vi "SQLite Insert or Update SensorConfigValue.vi"(7 "Main":string="0", 8 "error in (no error)":errorcluster, 9 "SensorConfigList":string, 11 "SensorName":string) -> (0 "error out":errorcluster, 3 "OK？":bool)   [LabVIEW 2017, in "SQLite.lvclass"]
doc: "保存传感器配置到Calibration.db.\n2020-03-06 09:56:51\n蒋松\njiangsong@outlook.com"
uses:
  SQLite.lvclass
  SQLiteFileName.ctl
  TabelFullName.ctl
  <vilib>/Utility/error.llb/Trim Whitespace.vi
  <userlib>/sushu/sushu.lvlib
  <userlib>/LabSQL/LabSQL.lvlib
panel:
  out "Insert DB String":string
  out "Insert DB String 2":string
  out "empty?":bool
  out "Select SQL CMD":string
  out "String":string
  in  "error in (no error) 2":errorcluster
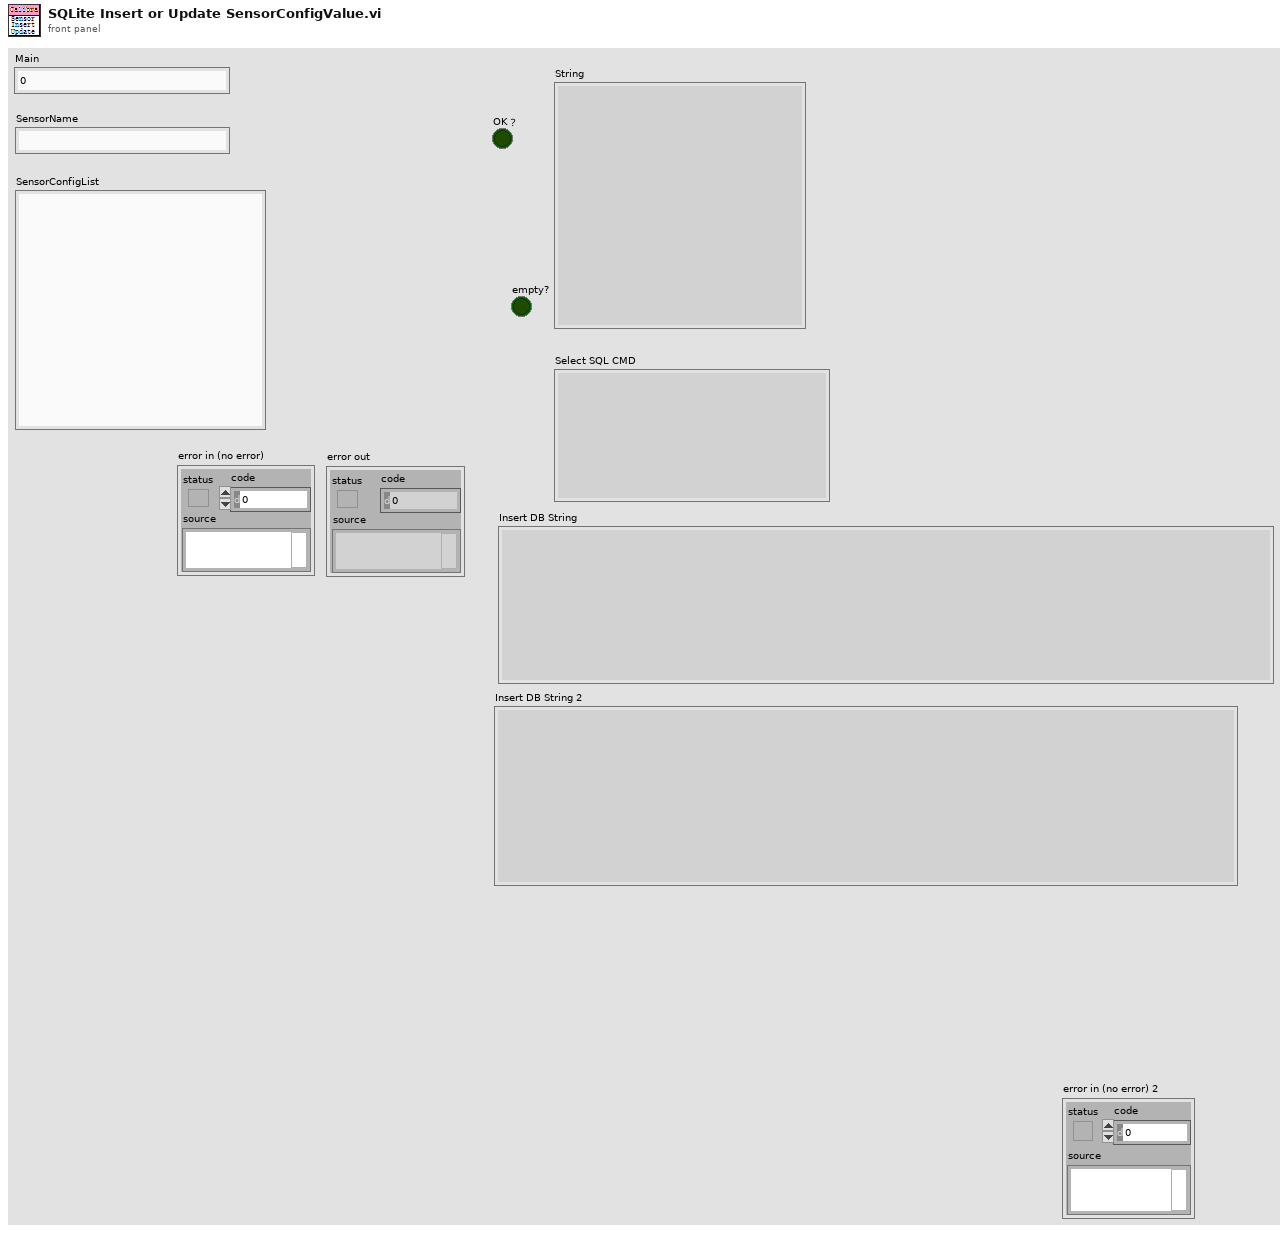
[diagram p1: front panel]
types:
  T1 = typedef "SQLite.lvclass/TabelFullName.ctl" = string
  T2 = typedef "SQLite.lvclass/SQLiteFileName.ctl" = string
  T3 = enum16{"Other", "SQL2008", "SQLite", "Access", "MySQL"}
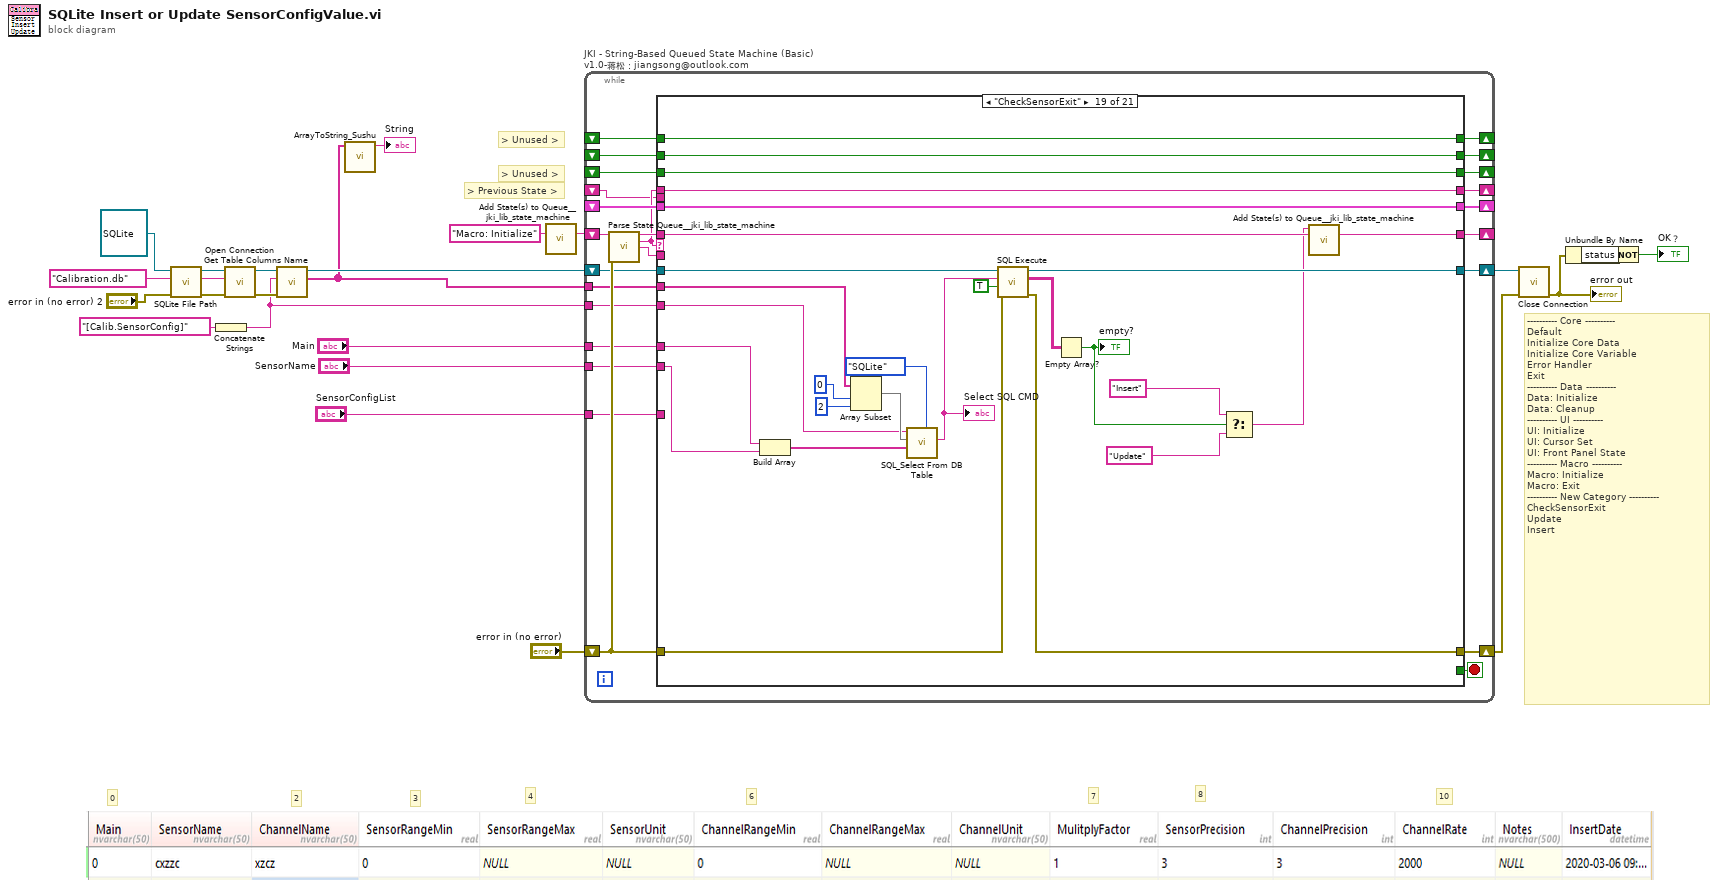
[diagram p0: block diagram]
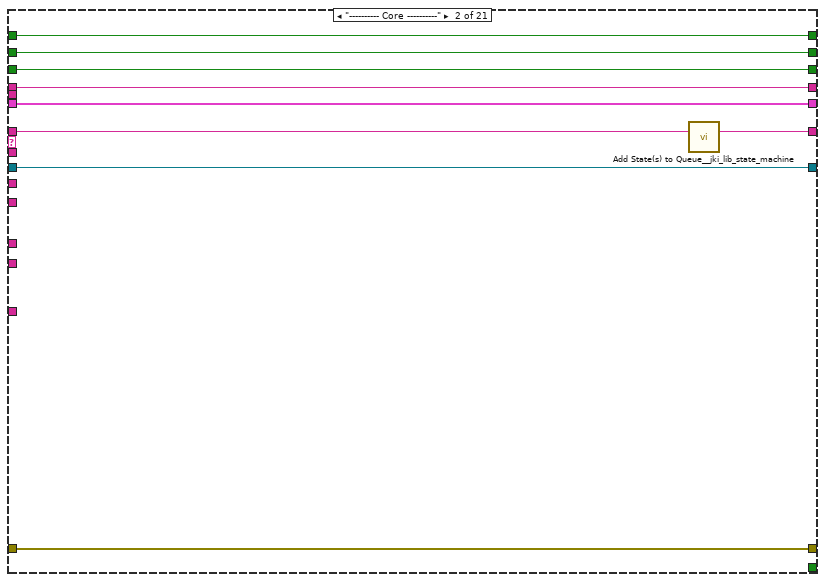
[diagram p3: hidden frame]
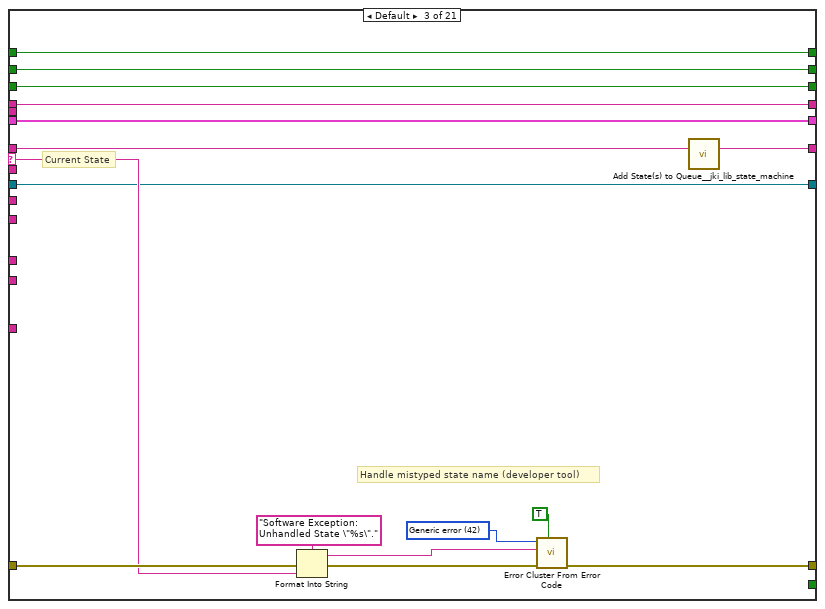
[diagram p4: hidden frame]
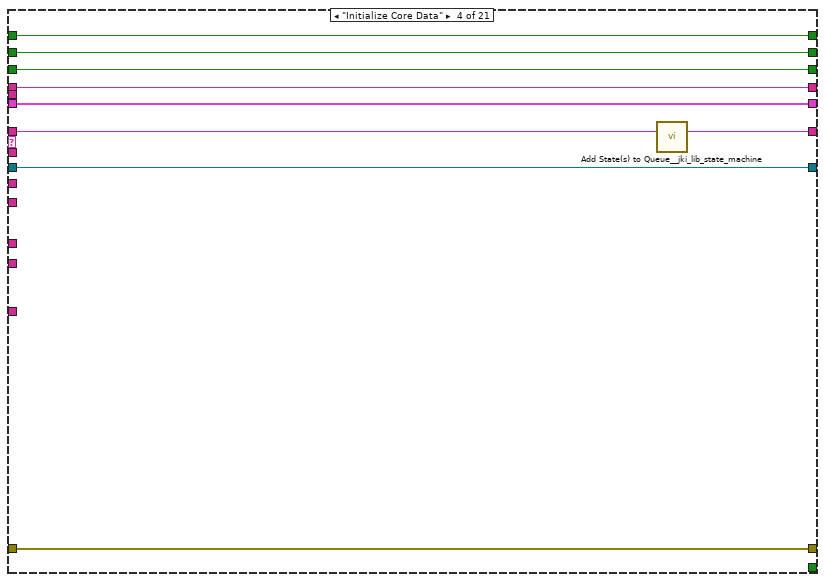
[diagram p5: hidden frame]
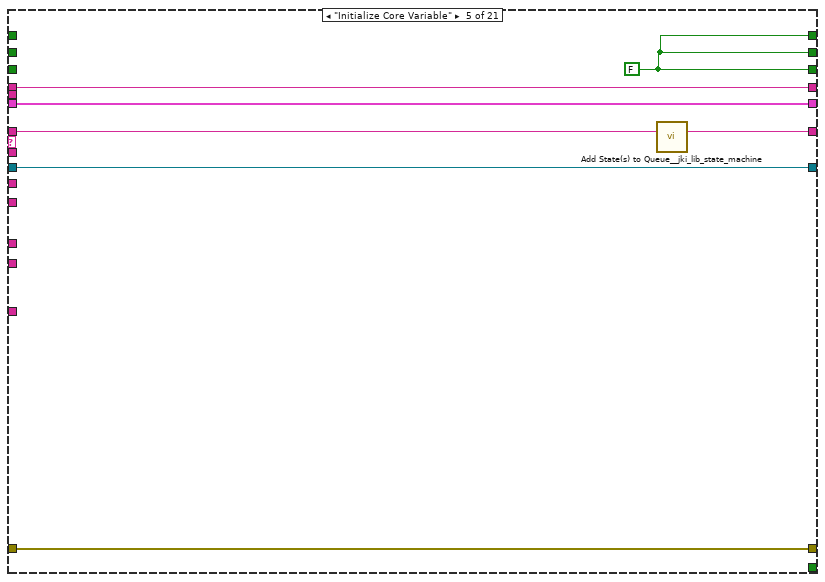
[diagram p6: hidden frame]
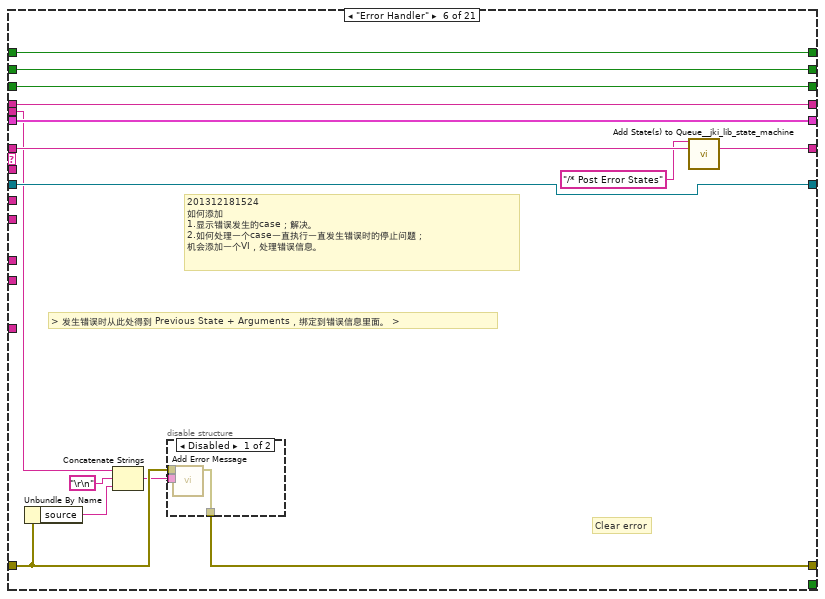
[diagram p7: hidden frame]
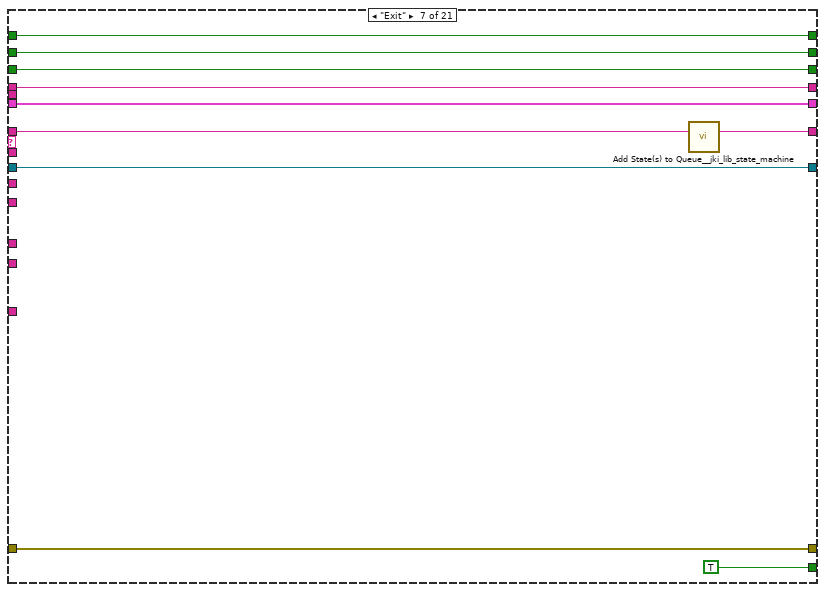
[diagram p9: hidden frame]
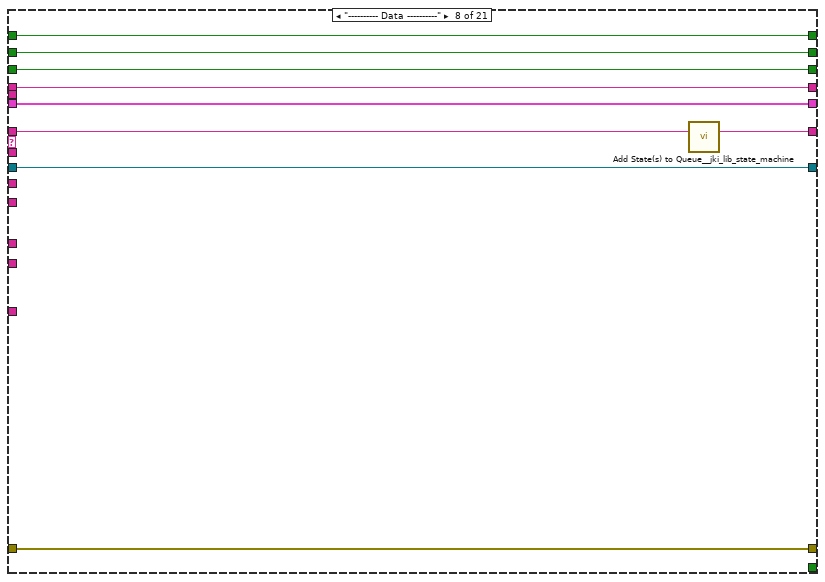
[diagram p10: hidden frame]
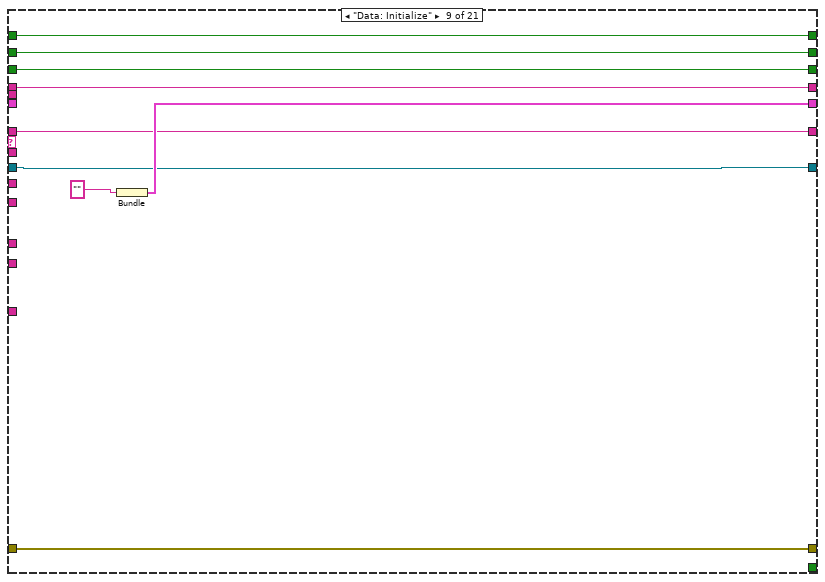
[diagram p11: hidden frame]
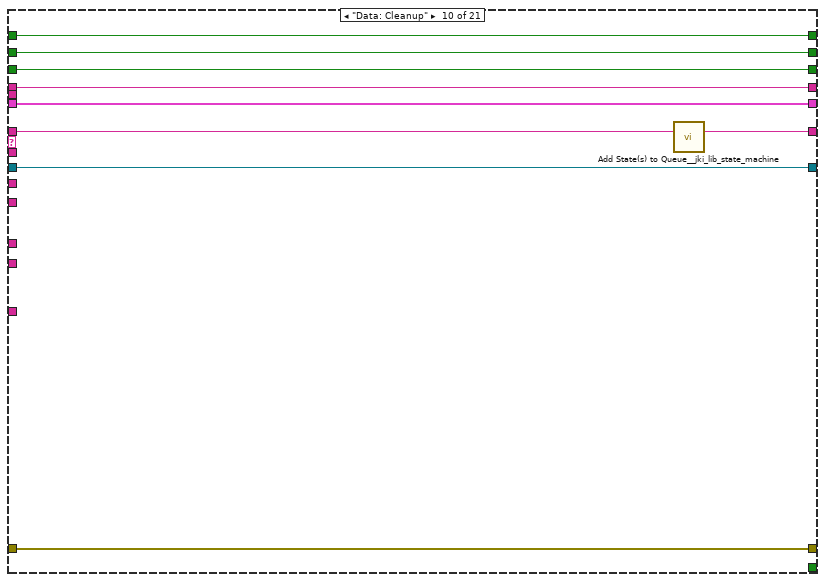
[diagram p12: hidden frame]
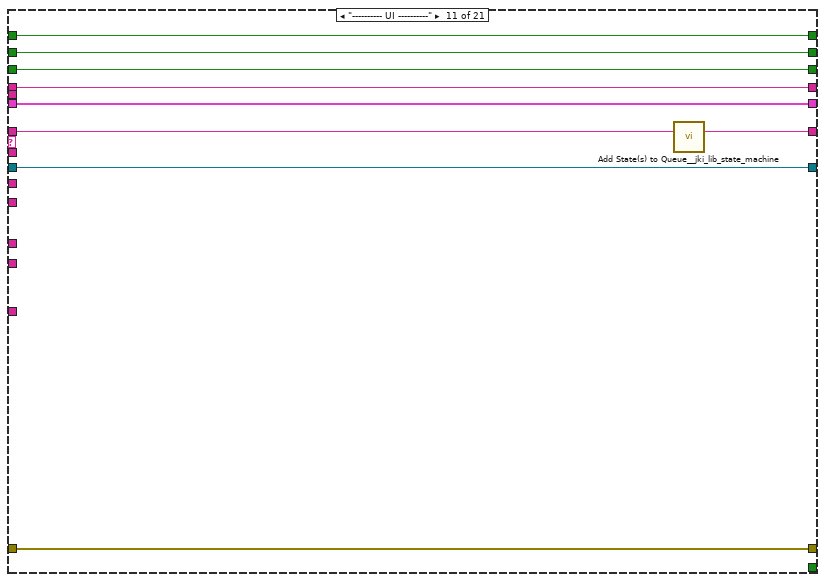
[diagram p13: hidden frame]
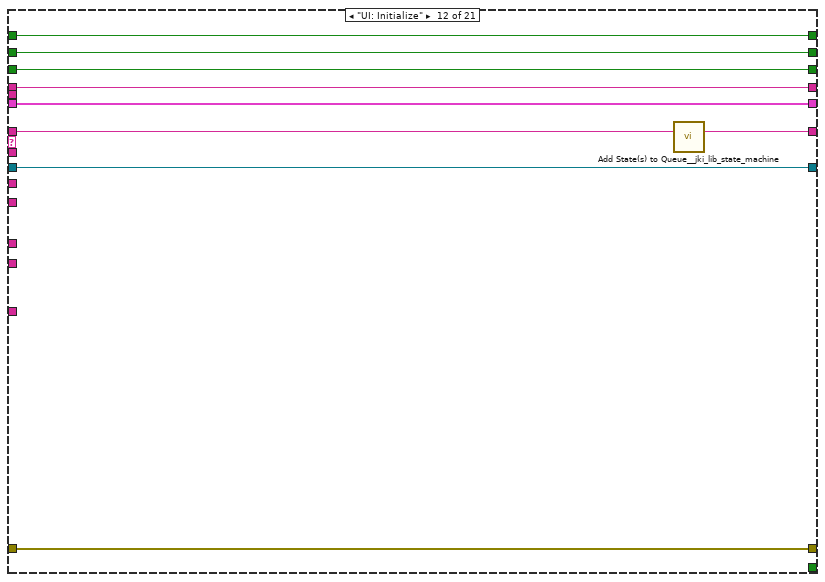
[diagram p14: hidden frame]
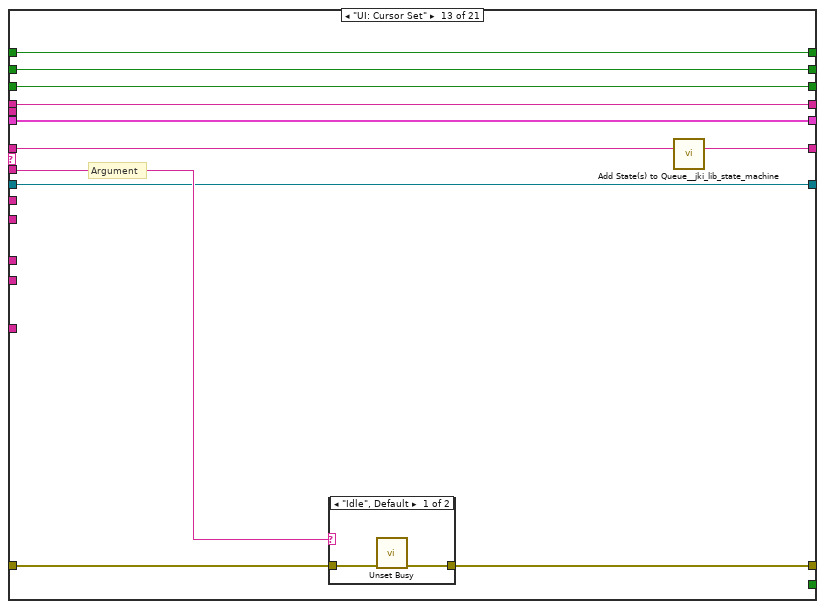
[diagram p15: hidden frame]
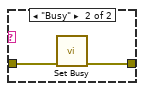
[diagram p16: hidden frame]
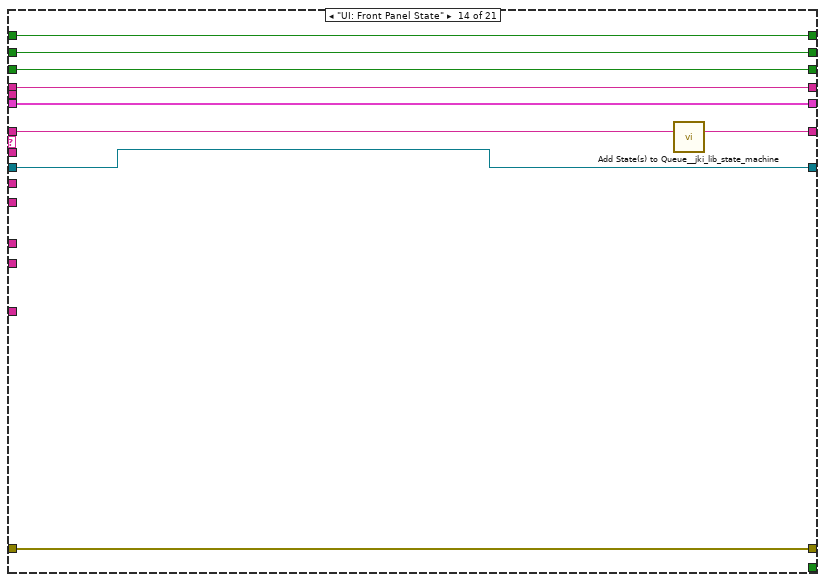
[diagram p17: hidden frame]
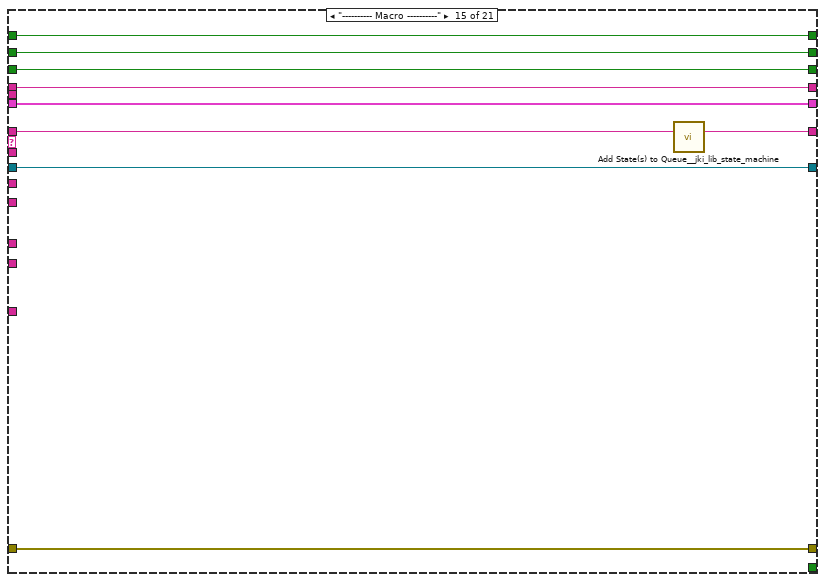
[diagram p18: hidden frame]
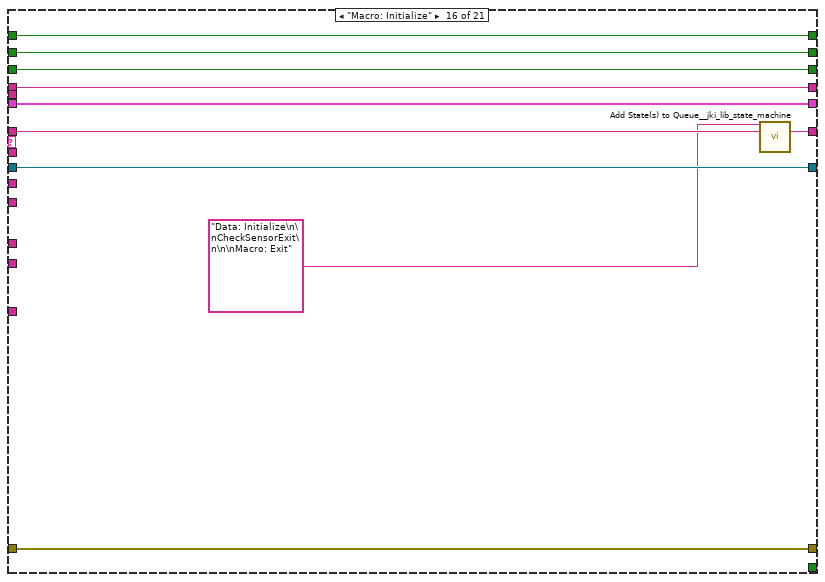
[diagram p19: hidden frame]
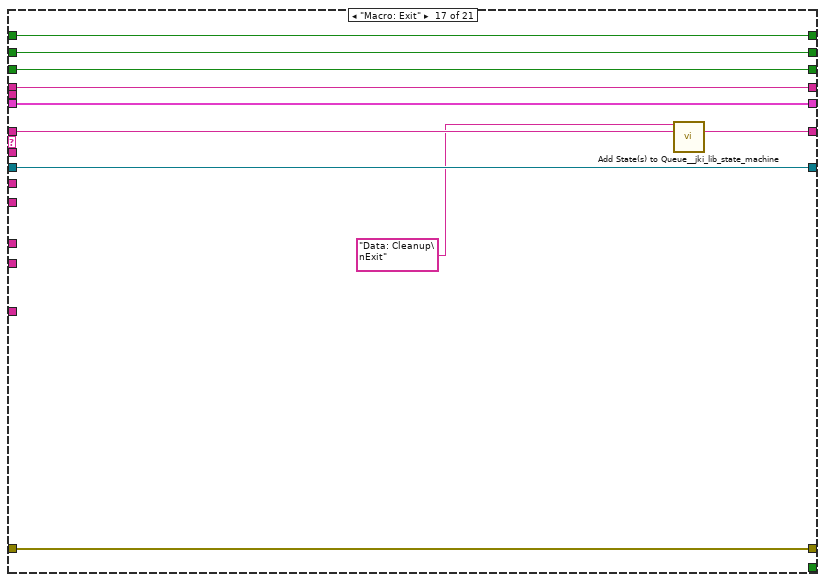
[diagram p20: hidden frame]
diagram:
  # "10"
  # "8"
  # "7"
  # "6"
  # "3"
  # "0"
  # "> Previous State >"
  # "> Unused >"
  # "> Unused >"
  # "---------- Core ----------\nDefault\nInitialize Core Data\nInitialize Core Variable\nError Handler\nExit\n---------- Data ----------\nData: Initialize\nData: Cleanup\n---------- UI ----------\nUI: Initialize\nUI: Cursor Set\nUI: Front Panel State\n---------- Macro ----------\nMacro: Initialize\nMacro: Exit\n---------- New Category ----------\nCheckSensorExit\nUpdate\nInsert"
  # "2"
  # "4"
  n1 = call "SQLite File Path.vi"("error in (no error)"="error in (no error) 2", "SQLiteFileName"=T2 "Calibration.db", "SQLite in"=refnum<class "SQLite.lvclass"> refnum ("SQLite.lvclass")) -> ("error out"=w19:errorcluster, "string"=w15:string, "SQLite out"=w17:refnum<class "SQLite.lvclass">)  [unwired: 6 in]
  n2 = Concatenate Strings(T1 "[Calib.SensorConfig]" ("TabelFullName")) -> (w10:string)
  n3 = call-dynamic "Open Connection.vi"("error in (no error)"=w19, "ConnectionString"=w15, "HostDB in"=w17) -> ("error out"=w14:errorcluster, "HostDB out"=w13:refnum<class "SQLite.lvclass">)  [unwired: 7 in]
  n4 = call-dynamic "Get Table Columns Name.vi"("error in (no error)"=w14, "TableName"=w10, "HostDB in"=w13) -> ("ColunmsList"=w6:string[], "HostDB out"=w11:refnum<class "SQLite.lvclass">)  [unwired: 4 in, 3 out]
  n5 = call <userlib>:"ArrayToString_Sushu.vi"("Array"=w6) -> ("String"=→"String":string)  [unwired: 10 in]
  n6 = call <vilib>:"Add State(s) to Queue__jki_lib_state_machine.vi"("State(s) in (\"\")"="Macro: Initialize") -> ("States Out"=w24:string)  [unwired: 14 in]
  n7 = while "JKI - String-Based Queued State Machine (Basic) v1.0-蒋松：jiangsong@outlook.com" {
    shift-right: [w47] -> w7
    shift-left: "error in (no error)" -> [w45]
    shift-right: [w28] -> _
    shift-left: w24 -> [w35]
    shift-right: [w41] -> _
    shift-left: _ -> [w43]
    shift-right: [w42] -> _
    shift-left: _ -> [w44]
    shift-right: [w36] -> _
    shift-left: _ -> [w39]
    shift-right: [w37] -> _
    shift-left: _ -> [w25]
    shift-right: [w38] -> _
    shift-left: _ -> [w40]
    tunnel: w6 -> [w34]
    tunnel: w10 -> [w33]
    tunnel: "Main" -> [w32]
    tunnel: "SensorName" -> [w31]
    shift-right: [w29] -> w9
    shift-left: w11 -> [w30]
    tunnel: "SensorConfigList" -> [w27]
    stop <- w46 stop-if-true
    n8 = call <vilib>:"Parse State Queue__jki_lib_state_machine.vi"("State Queue"=w35, "Error In (no error)"=w45) -> ("Remaining States"=w49:string, "Current State"=w26:string, "Arguments"=w48:string)  [unwired: 10 in, 1 out]
    n9 = case shown="\"CheckSensorExit\"" w26 {
      selector: w26 -> [_ _ w68 _ _ _ _ _ _ _ _ _ _ _ _ _ _ _ _ _ _]
      tunnel: w49 -> [w50 w66 w82 w91 w98 w113 w126 w135 w136 w153 w162 w171 w182 w195 w204 w206 w224 w233 w239 w283 w311]
      tunnel: w48 -> [_ _ _ _ _ _ _ _ _ _ _ _ w176 _ _ _ _ _ _ _ _]
      tunnel: [w57 w64 w69 w86 w96 w100 w119 w129 w141 w145 w156 w165 w174 w187 w198 w210 w219 w228 w236 w261 w285] -> w47
      tunnel: w45 -> [w57 w64 w70 w86 w96 w103 w119 w129 w141 w145 w156 w165 w175 w187 w198 w210 w219 w228 w237 w262 w286]
      tunnel: [w50 w65 w81 w90 w97 w112 w125 w134 w136 w152 w161 w170 w181 w194 w203 w207 w223 w232 w240 w283 w311] -> w28
      tunnel: [_ _ _ _ _ _ TRUE _ _ _ _ _ _ _ _ _ _ _ _ _ _] -> w46
      tunnel: w44 -> [w56 w63 w80 w89 _ w111 w124 w133 w144 w151 w160 w169 w180 w193 w202 w214 w222 w231 w260 w282 w310]
      tunnel: w43 -> [w55 w62 w79 w88 _ w110 w123 w132 w143 w150 w159 w168 w179 w192 w201 w213 w221 w230 w259 w281 w309]
      tunnel: [w56 w63 w80 w89 w93 w111 w124 w133 w144 w151 w160 w169 w180 w193 w202 w214 w222 w231 w260 w282 w310] -> w42
      tunnel: [w55 w62 w79 w88 w93 w110 w123 w132 w143 w150 w159 w168 w179 w192 w201 w213 w221 w230 w259 w281 w309] -> w41
      tunnel: w40 -> [w54 w61 w78 w87 _ w109 w122 w131 w142 w149 w158 w167 w178 w191 w200 w212 w220 w229 w258 w280 w308]
      tunnel: w26 -> [w52 w59 w77 w85 w92 w106 w118 w128 w139 w147 w155 w164 w173 w189 w197 w209 w217 w226 w257 w279 w307]
      tunnel: w39 -> [w53 w60 w76 w83 w95 w101 w121 w130 _ w148 w157 w166 w177 w190 w199 w211 w218 w227 w256 w278 w306]
      tunnel: [w54 w61 w78 w87 w93 w109 w122 w131 w142 w149 w158 w167 w178 w191 w200 w212 w220 w229 w258 w280 w308] -> w38
      tunnel: [w52 w59 w77 w85 w92 w106 w118 w128 w139 w147 w155 w164 w173 w189 w197 w209 w217 w226 w257 w279 w307] -> w37
      tunnel: [w53 w60 w76 w83 w95 w101 w121 w130 w140 w148 w157 w166 w177 w190 w199 w211 w218 w227 w256 w278 w306] -> w36
      tunnel: w34 -> [_ _ _ _ _ _ _ _ _ _ _ _ _ _ _ _ _ _ w247 w270 w292]
      tunnel: w33 -> [_ _ _ _ _ _ _ _ _ _ _ _ _ _ _ _ _ _ w246 w272 w299]
      tunnel: w32 -> [_ _ _ _ _ _ _ _ _ _ _ _ _ _ _ _ _ _ w245 w277 w305]
      tunnel: w31 -> [_ _ _ _ _ _ _ _ _ _ _ _ _ _ _ _ _ _ w244 w276 w304]
      tunnel: w30 -> [w51 w58 w67 w84 w94 w104 w117 w127 w138 w146 w154 w163 w172 w188 w196 w208 w216 w225 w249 w275 w303]
      tunnel: [w51 w58 w67 w84 w94 w104 w117 w127 w138 w146 w154 w163 w172 w188 w196 w208 w216 w225 w248 w274 w302] -> w29
      tunnel: w27 -> [_ _ _ _ _ _ _ _ _ _ _ _ _ _ _ _ _ _ _ w267 w296]
      tunnel: w25 -> [_ _ _ _ _ w99 _ _ _ _ _ _ _ _ _ _ _ _ _ _ _]
      frame "Idle" {
      }
      frame "---------- Core ----------" {
        n10 = call <vilib>:"Add State(s) to Queue__jki_lib_state_machine.vi"("State(s) in (\"\")"=w66) -> ("States Out"=w65:string)  [unwired: 14 in]
      }
      frame Default {
        w72 = 42 items=["No error", "Argument error", "Memory is full", "Out of zone", "End of file", "File already open", "Generic file I/O error", "File not found", "File permission error", "Disk is full", "Duplicate path", "Too many files open", "System feature not enabled", "Resource file not found", "Cannot add resource", "Resource not found", "Image not found", "Image memory error", "Pen does not exist", "Config type invalid", "Config token not found", "Config parse error", "Config memory error", "Bad external code format", "Bad external code offset", "External code not present", "Null window", "Destroy window error", "Null menu", "Print aborted", "Bad print record", "Print driver error", "Windows error during printing", "Memory error during printing", "Print dialog error", "Generic print error", "Invalid device refnum", "Device not found", "Device parameter error", "Device unit error", "Cannot open device", "Device call aborted", "Generic error", "Cancelled by user", "Object ID too low", "Object ID too high", "Object not in heap", "Unknown heap", "Unknown object (invalid DefProc)", "Unknown object (DefProc not in table)", "Message out of range", "Invalid (null) method", "Unknown message", "Manager call not supported", "Bad address", "Network operation in progress", "Network operation timed out", "Connection is busy", "Network attribute not supported", "Network error", "Address in use", "System out of memory", "Connection aborted", "Connection refused", "Not connected", "Already connected", "Connection closed", "Initialization error (interapplication manager)", "Bad occurrence", "Wait on unbound occurrence handler", "Occurrence queue overflow", "Datalog type conflict", "Unused", "Unrecognized type (interapplication manager)", "Memory corrupt", "Failed to make temporary DLL", "Old CIN version", "Drag socket not found", "Failed to load drop-object", "Failed to register OLE object", "Failed to release OLE object", "Format specifier type mismatch", "Unknown format specifier", "Too few format specifiers", "Too many format specifiers", "Scan failed", "Newer CIN version", "Error converting to variant", "Runtime menu error", "Password tampered", "Variant attribute not found", "Incompatible variant data type", "Event data is not available", "Event Store is not present", "Occurrence is not found", "Event Queue is not created", "Event info is not available", "Refnum passed is NULL", "Error retrieving Class GUID", "Error retrieving CoClass GUID", "Error retrieving TypeLib GUID.", "Bad built application magic bytes.", "Specific driver is different from the specific driver associated with the Logical Name.", "There is no session opened to the class driver.", "Max Error", "MAX - Error with config objects", "MAX - Error loading configuration", "MAX - Group not supported"]
        # "Current State"
        # "Handle mistyped state name (developer tool)"
        n11 = Format Into String(format string="Software Exception: Unhandled State \"%s\"." ("message"), error in=w70, w68) -> (resulting string=w73:string, error out=w74:errorcluster)  [unwired: 1 in]
        n12 = call <vilib>:"Error Cluster From Error Code.vi"("show call chain? (False)"=TRUE, "error in (no error)"=w74, "error message (\"\")"=w73, "error code (0)"=w72) -> ("error out"=w69:errorcluster)  [unwired: 5 in]
        n13 = call <vilib>:"Add State(s) to Queue__jki_lib_state_machine.vi"("State(s) in (\"\")"=w82) -> ("States Out"=w81:string)  [unwired: 14 in]
      }
      frame "Initialize Core Data" {
        n14 = call <vilib>:"Add State(s) to Queue__jki_lib_state_machine.vi"("State(s) in (\"\")"=w91) -> ("States Out"=w90:string)  [unwired: 14 in]
      }
      frame "Initialize Core Variable" {
        w93 = FALSE
        n15 = call <vilib>:"Add State(s) to Queue__jki_lib_state_machine.vi"("State(s) in (\"\")"=w98) -> ("States Out"=w97:string)  [unwired: 14 in]
      }
      frame "Error Handler" {
        # "> 发生错误时从此处得到 Previous State + Arguments，绑定到错误信息里面。 >"
        # "201312181524\n如何添加\n1.显示错误发生的case；解决。\n2.如何处理一个case一直执行一直发生错误时的停止问题；\n机会添加一个VI，处理错误信息。"
        # "Clear error"
        n16 = Unbundle By Name(w103) -> ("source"=w105:string)
        n17 = Concatenate Strings(w99, "\r\n", w105) -> (w102:string)
        n18 = disable-structure shown="Disabled" {
          disable-tunnel: w103 -> [w116 _]
          disable-tunnel: w102 -> [w115 _]
          disable-tunnel: [w114 _] -> w100
          frame Disabled {
            n19 = call <userlib>:"Add Error Message.vi"("ErrorMessages"=w115, "error in (no error)"=w116) -> ("error out"=w114:errorcluster)  [unwired: 9 in]
          }
          frame Enabled {
          }
        }
        n20 = call <vilib>:"Add State(s) to Queue__jki_lib_state_machine.vi"("State(s) in Front (\"\")"="/* Post Error States", "State(s) in (\"\")"=w113) -> ("States Out"=w112:string)  [unwired: 13 in]
      }
      frame "Exit" {
        n21 = call <vilib>:"Add State(s) to Queue__jki_lib_state_machine.vi"("State(s) in (\"\")"=w126) -> ("States Out"=w125:string)  [unwired: 14 in]
      }
      frame "---------- Data ----------" {
        n22 = call <vilib>:"Add State(s) to Queue__jki_lib_state_machine.vi"("State(s) in (\"\")"=w135) -> ("States Out"=w134:string)  [unwired: 14 in]
      }
      frame "Data: Initialize" {
        n23 = Bundle("") -> (w140:cluster{string})  [unwired: 1 in]
      }
      frame "Data: Cleanup" {
        n24 = call <vilib>:"Add State(s) to Queue__jki_lib_state_machine.vi"("State(s) in (\"\")"=w153) -> ("States Out"=w152:string)  [unwired: 14 in]
      }
      frame "---------- UI ----------" {
        n25 = call <vilib>:"Add State(s) to Queue__jki_lib_state_machine.vi"("State(s) in (\"\")"=w162) -> ("States Out"=w161:string)  [unwired: 14 in]
      }
      frame "UI: Initialize" {
        n26 = call <vilib>:"Add State(s) to Queue__jki_lib_state_machine.vi"("State(s) in (\"\")"=w171) -> ("States Out"=w170:string)  [unwired: 14 in]
      }
      frame "UI: Cursor Set" {
        # "Argument"
        n27 = case shown="\"Idle\", Default" w176 {
          tunnel: w175 -> [w184 w186]
          tunnel: [w183 w185] -> w174
          frame "Idle", Default {
            n28 = call <vilib>:"Unset Busy.vi"("error in (no error)"=w184) -> ("error out"=w183:errorcluster)  [unwired: 10 in]
          }
          frame "Busy" {
            n29 = call <vilib>:"Set Busy.vi"("error in (no error)"=w186) -> ("error out"=w185:errorcluster)  [unwired: 9 in, 1 out]
          }
        }
        n30 = call <vilib>:"Add State(s) to Queue__jki_lib_state_machine.vi"("State(s) in (\"\")"=w182) -> ("States Out"=w181:string)  [unwired: 14 in]
      }
      frame "UI: Front Panel State" {
        n31 = call <vilib>:"Add State(s) to Queue__jki_lib_state_machine.vi"("State(s) in (\"\")"=w195) -> ("States Out"=w194:string)  [unwired: 14 in]
      }
      frame "---------- Macro ----------" {
        n32 = call <vilib>:"Add State(s) to Queue__jki_lib_state_machine.vi"("State(s) in (\"\")"=w204) -> ("States Out"=w203:string)  [unwired: 14 in]
      }
      frame "Macro: Initialize" {
        n33 = call <vilib>:"Add State(s) to Queue__jki_lib_state_machine.vi"("State(s) in Front (\"\")"="Data: Initialize\n\nCheckSensorExit\n\n\nMacro: Exit", "State(s) in (\"\")"=w206) -> ("States Out"=w207:string)  [unwired: 13 in]
      }
      frame "Macro: Exit" {
        n34 = call <vilib>:"Add State(s) to Queue__jki_lib_state_machine.vi"("State(s) in Front (\"\")"="Data: Cleanup\nExit", "State(s) in (\"\")"=w224) -> ("States Out"=w223:string)  [unwired: 13 in]
      }
      frame "---------- New Category ----------" {
        n35 = call <vilib>:"Add State(s) to Queue__jki_lib_state_machine.vi"("State(s) in (\"\")"=w233) -> ("States Out"=w232:string)  [unwired: 14 in]
      }
      frame "CheckSensorExit" {
        n36 = Build Array(w245, w244) -> (w253:string[])
        n37 = Array Subset(array=w247, index=0, length=2) -> (w251:string[])
        n38 = call <userlib>:"SQL_Select From DB Table.vi"("DB Type"=T3."SQLite", "ColumnsValue"=w253, "ColumnsNameList"=w251, "TableName"=w246) -> ("Select SQL CMD"=w254:string)  [unwired: 7 in]
        "Select SQL CMD" <- w254
        n39 = call-dynamic "SQL Execute.vi"("error in (no error)"=w237, "Return Data (T)"=TRUE, "Command Text"=w254, "HostDB in"=w249) -> ("error out"=w236:errorcluster, "Table Control"=w255:string[][], "HostDB out"=w248:refnum<class "SQLite.lvclass">)  [unwired: 3 in, 2 out]
        n40 = Empty Array?(array=w255) -> (empty?=w243:bool)
        "empty?" <- w243
        n41 = Select(t="Insert", s=w243, f="Update") -> (s? t:f=w238:string)
        n42 = call <vilib>:"Add State(s) to Queue__jki_lib_state_machine.vi"("State(s) in Front (\"\")"=w238, "State(s) in (\"\")"=w239) -> ("States Out"=w240:string)  [unwired: 13 in]
      }
      frame "Insert" {
        n43 = call <userlib>:"StringToArray_Sushu.vi"("State Queue"=w267) -> ("Array"=w266:string[])  [unwired: 8 in, 2 out]
        n44 = Build Array (concatenate)(w277, w276, w266) -> (w265:string[])
        n45 = Array Size(array=w265) -> (size(s)=w264:i32)
        n46 = Array Subset(array=w270, index=0, length=w264) -> (w271:string[])
        n47 = call <userlib>:"SQL_Insert DB Table.vi"("DB Type"=enum16{"Other", "SQL2008", "SQLite"}."SQLite", "ColumnsValue"=w265, "ColumnsName"=w271, "Table Name"=w272) -> ("Insert DB String"=w263:string)  [unwired: 7 in]
        "Insert DB String" <- w263
        n48 = call-dynamic "SQL Execute.vi"("error in (no error)"=w262, "Return Data (T)"=FALSE, "Command Text"=w263, "HostDB in"=w275) -> ("error out"=w261:errorcluster, "HostDB out"=w274:refnum<class "SQLite.lvclass">)  [unwired: 3 in, 3 out]
      }
      frame "Update" {
        (unwired) enum16{"Other", "SQL2008", "SQLite"}."SQLite" ("DB Type")
        n49 = call <userlib>:"StringToArray_Sushu.vi"("State Queue"=w296) -> ("Array"=w287:string[])  [unwired: 8 in, 2 out]
        n50 = Build Array(w305, w304) -> (w294:string[])
        n51 = Array Subset(array=w292, index=0, length=2) -> (w290:string[])
        n52 = Array Size(array=w287) -> (size(s)=w295:i32)
        n53 = call <userlib>:"Build string_ColumnsName=ColumnsValue_Where and.vi"("DB Type"=T3."SQLite", "ColumnsValue"=w294, "Check ASCII?"=FALSE, "ColumnsNameList"=w290) -> ("ColumnName='ColumnValue'"=w288:string)  [unwired: 7 in]
        n54 = Array Subset(array=w292, index=2, length=w295) -> (w298:string[])
        n55 = call <userlib>:"SQL_Update DB Table.vi"("where name='value'"=w288, "ColumnsValue"=w287, "ColumnsNameList"=w298, "TableName"=w299) -> ("Update CMD"=w300:string)  [unwired: 7 in]
        "Insert DB String 2" <- w300
        n56 = call-dynamic "SQL Execute.vi"("error in (no error)"=w286, "Return Data (T)"=FALSE, "Command Text"=w300, "HostDB in"=w303) -> ("error out"=w285:errorcluster, "HostDB out"=w302:refnum<class "SQLite.lvclass">)  [unwired: 3 in, 3 out]
      }
    }
  }
  n57 = call-dynamic "Close Connection.vi"("error in (no error)"=w7, "HostDB in"=w9) -> ("error out"=w3:errorcluster)  [unwired: 8 in, 1 out]
  "error out" <- w3
  n58 = Unbundle By Name(w3) -> ("status"=w2:bool)
  n59 = Not(x=w2) -> (.not. x?=→"OK？":bool)
